vi "All_Off_Relays.vi"() -> (0 "error out":errorcluster)   [LabVIEW 2023]
uses:
  <vilib>/ULx/Create Channel.llb/ULx Create Channel (DO-Digital Output).vi
  <vilib>/ULx/Write.llb/ULx Write (Digital 1D Bool 1Chan 1Samp).vi
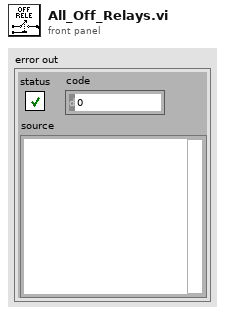
[diagram p1: front panel]
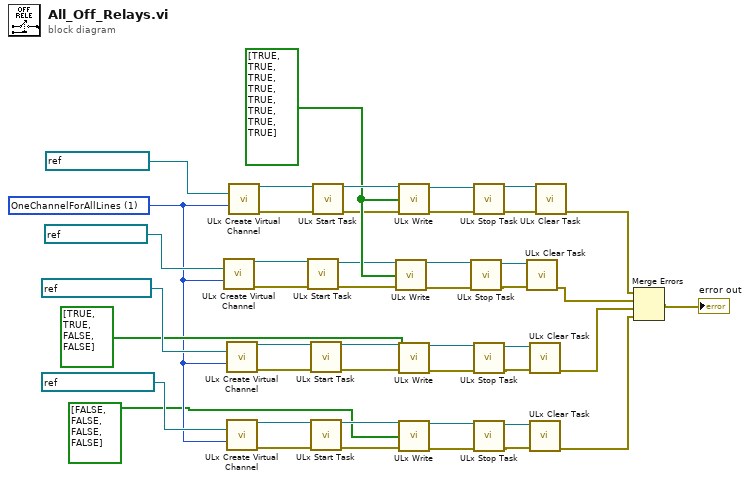
[diagram p0: block diagram]
diagram:
  w8 = 1 items=["OneChannelForEachLine", "OneChannelForAllLines"] ("line grouping")
  w39 = bool[] [TRUE, TRUE, TRUE, TRUE, TRUE, TRUE, TRUE, TRUE] ("data")
  n1 = call-poly <vilib>:"ULx Create Virtual Channel.vi"("lines"=refnum<k21> "Dev0/1stPortB", "line grouping"=w8) -> ("task out"=w32:refnum<k24>, "error out"=w31:errorcluster)  [unwired: 12 in]
  n2 = call-poly <vilib>:"ULx Create Virtual Channel.vi"("lines"=refnum<k21> "Dev0/1stPortCL", "line grouping"=w8) -> ("task out"=w24:refnum<k24>, "error out"=w23:errorcluster)  [unwired: 12 in]
  n3 = call-poly <vilib>:"ULx Create Virtual Channel.vi"("lines"=refnum<k21> "Dev0/1stPortCH", "line grouping"=w8) -> ("task out"=w14:refnum<k24>, "error out"=w13:errorcluster)  [unwired: 12 in]
  n4 = call-poly <vilib>:"ULx Create Virtual Channel.vi"("lines"=refnum<k21> "Dev0/1stPortA", "line grouping"=w8) -> ("task out"=w44:refnum<k24>, "error out"=w45:errorcluster)  [unwired: 12 in]
  n5 = call <vilib>:"ULx Start Task.vi"("task in"=w32, "error in"=w31) -> ("task out"=w7:refnum<k24>, "error out"=w30:errorcluster)  [unwired: 12 in]
  n6 = call <vilib>:"ULx Start Task.vi"("task in"=w24, "error in"=w23) -> ("task out"=w21:refnum<k24>, "error out"=w22:errorcluster)  [unwired: 12 in]
  n7 = call <vilib>:"ULx Start Task.vi"("task in"=w14, "error in"=w13) -> ("task out"=w11:refnum<k24>, "error out"=w12:errorcluster)  [unwired: 12 in]
  n8 = call <vilib>:"ULx Start Task.vi"("task in"=w44, "error in"=w45) -> ("task out"=w43:refnum<k24>, "error out"=w38:errorcluster)  [unwired: 12 in]
  n9 = call-poly <vilib>:"ULx Write.vi"("task in"=w7, "data"=w39, "error in"=w30) -> ("task out"=w36:refnum<k24>, "error out"=w35:errorcluster)  [unwired: 10 in, 1 out]
  n10 = call-poly <vilib>:"ULx Write.vi"("task in"=w43, "data"=w39, "error in"=w38) -> ("task out"=w20:refnum<k24>, "error out"=w41:errorcluster)  [unwired: 10 in, 1 out]
  n11 = call-poly <vilib>:"ULx Write.vi"("task in"=w21, "data"=bool[] [TRUE, TRUE, FALSE, FALSE], "error in"=w22) -> ("task out"=w28:refnum<k24>, "error out"=w27:errorcluster)  [unwired: 10 in, 1 out]
  n12 = call-poly <vilib>:"ULx Write.vi"("task in"=w11, "data"=bool[] [FALSE, FALSE, FALSE, FALSE], "error in"=w12) -> ("task out"=w18:refnum<k24>, "error out"=w17:errorcluster)  [unwired: 10 in, 1 out]
  n13 = call <vilib>:"ULx Stop Task.vi"("error in"=w35, "task in"=w36) -> ("error out"=w33:errorcluster, "task out"=w34:refnum<k24>)  [unwired: 8 in]
  n14 = call <vilib>:"ULx Stop Task.vi"("error in"=w41, "task in"=w20) -> ("error out"=w42:errorcluster, "task out"=w19:refnum<k24>)  [unwired: 8 in]
  n15 = call <vilib>:"ULx Stop Task.vi"("error in"=w27, "task in"=w28) -> ("error out"=w25:errorcluster, "task out"=w26:refnum<k24>)  [unwired: 8 in]
  n16 = call <vilib>:"ULx Stop Task.vi"("error in"=w17, "task in"=w18) -> ("error out"=w15:errorcluster, "task out"=w16:refnum<k24>)  [unwired: 8 in]
  n17 = call <vilib>:"ULx Clear Task.vi"("task in"=w34, "error in"=w33) -> ("error out"=w4:errorcluster)  [unwired: 13 in]
  n18 = call <vilib>:"ULx Clear Task.vi"("task in"=w26, "error in"=w25) -> ("error out"=w3:errorcluster)  [unwired: 13 in]
  n19 = call <vilib>:"ULx Clear Task.vi"("task in"=w16, "error in"=w15) -> ("error out"=w2:errorcluster)  [unwired: 13 in]
  n20 = call <vilib>:"ULx Clear Task.vi"("task in"=w19, "error in"=w42) -> ("error out"=w5:errorcluster)  [unwired: 13 in]
  n21 = Merge Errors(w5, w4, w3, w2) -> (→"error out":errorcluster)
